vi "CameraAttributeTest.vi"() -> ()   [LabVIEW 2020]
uses:
  <vilib>/userDefined/High Color/IMAQdx.ctl
  <resource>/objmgr/imaqdx.rc
  <vilib>/vision/driver/NI_Vision_Acquisition_Software.lvlib
panel:
  in  "Trigger state":bool
  in  "Session In":T1
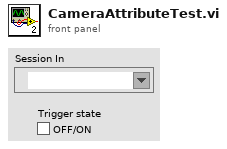
[diagram p1: front panel]
types:
  T1 = typedef "IMAQdx.ctl" = refnum<k21>
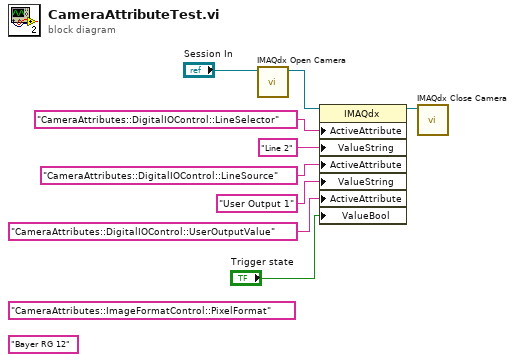
[diagram p0: block diagram]
diagram:
  (unwired) "Bayer RG 12" ("ValueString")
  (unwired) "CameraAttributes::ImageFormatControl::PixelFormat" ("ActiveAttribute")
  n1 = call <vilib>:"IMAQdx Open Camera.vi"("Session In"="Session In") -> ("Session Out"=w3:T1)  [unwired: 9 in, 1 out]
  n2 = property class="IMAQdx"(reference=w3, "ActiveAttribute"="CameraAttributes::DigitalIOControl::LineSelector", "ValueString"="Line 2", "ActiveAttribute"="CameraAttributes::DigitalIOControl::LineSource", "ValueString"="User Output 1", "ActiveAttribute"="CameraAttributes::DigitalIOControl::UserOutputValue", "ValueBool"="Trigger state") -> (reference out=w2:T1)  [unwired: 1 in, 1 out]
  n3 = call <vilib>:"IMAQdx Close Camera.vi"("Session In"=w2) -> ()  [unwired: 10 in, 1 out]
